vi "Sub Initialize.vi"(8 "error in (no error)":errorcluster, 11 "Instrument Recorder in":refnum<class "PID Controller.lvclass">) -> (0 "error out":errorcluster, 2 "Initialize Result":refnum<class "Acquired Result.lvclass">, 3 "Instrument Recorder out":refnum<class "PID Controller.lvclass">)   [LabVIEW 2018, in "PID Controller.lvclass"]
uses:
  PID Controller.lvclass
  C:/Program Files/National Instruments/LabVIEW 2018/vi.lib/ActorFramework/Actor/Actor.lvclass
  NHMFL_Core/Libraries/Instruments/Results/Acquired Result/Acquired Result.lvclass
  <vilib>/ActorFramework/Actor/Actor.lvclass/Actor.ctl
  <vilib>/ActorFramework/Message Enqueuer/Message Enqueuer.lvclass/Message Enqueuer.ctl
  Template Module Messages/Subscribe Request Msg/Subscribe Request Msg.lvclass/Subscribe Request Msg.ctl
  <vilib>/ActorFramework/Message Enqueuer/Init from Existing Queue.vi
  <vilib>/ActorFramework/Message Enqueuer/Enqueue.vi
  Template Module Messages/Subscribe Request Msg/Subscribe Request Msg.lvclass
  C:/Program Files/National Instruments/LabVIEW 2018/vi.lib/ActorFramework/Message/Message.lvclass
  <vilib>/ActorFramework/Message Priority Queue/Priority Enqueue.vi
  <vilib>/ActorFramework/Message Enqueuer/Message Enqueuer.lvclass
  Instrument Actor/Instrument Actor.lvclass
  <vilib>/ActorFramework/Actor/Actor.lvclass
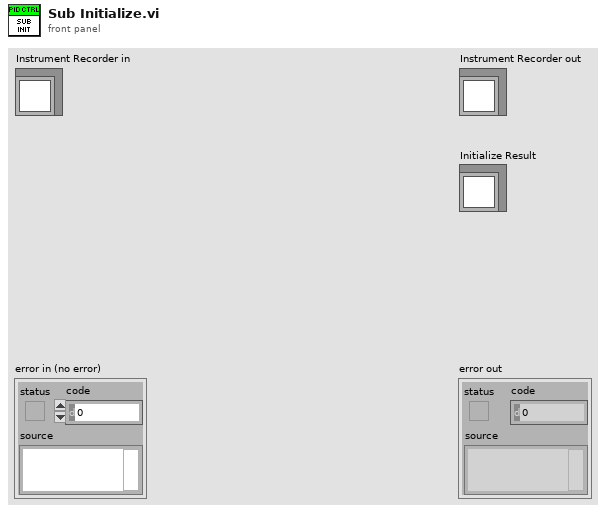
[diagram p1: front panel]
types:
  T1 = typedef "PID Controller Configuration.ctl" = cluster{"P":dbl, "I":dbl, "D":dbl, "Set point":dbl, "Input instrument":string, "Output instrument":string}
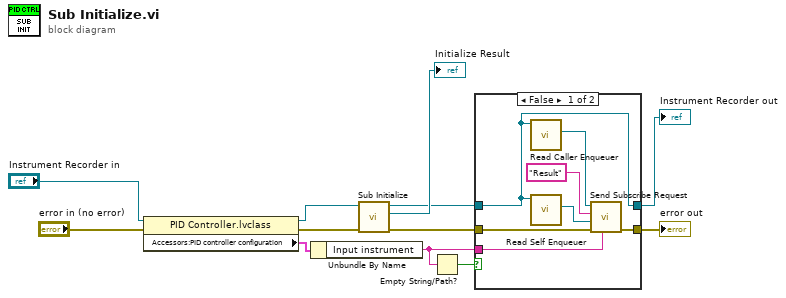
[diagram p0: block diagram]
diagram:
  n1 = property class="PID Controller.lvclass"(reference="Instrument Recorder in", error in="error in (no error)") -> (reference out=w1:refnum<class "PID Controller.lvclass">, error out=w2:errorcluster, "Accessors:PID controller configuration"=w9:T1)
  n2 = Unbundle By Name(w9) -> ("Input instrument"=w5:string)
  n3 = call-parent "Sub Initialize.vi"("error in (no error)"=w2, "Instrument Recorder in"=w1) -> ("error out"=w4:errorcluster, "Initialize Result"=→"Initialize Result":refnum<class "Acquired Result.lvclass">, "Instrument Recorder out"=w7:refnum<class "PID Controller.lvclass">)  [unwired: 7 in]
  n4 = Empty String/Path?(string/path=w5) -> (empty?=w8:bool)
  n5 = case shown="False" w8 {
    tunnel: w5 -> [w17 _]
    tunnel: w7 -> [w14 w21]
    tunnel: [w14 w21] -> w6
    tunnel: w4 -> [w19 w20]
    tunnel: [w18 w20] -> w3
    frame False {
      n6 = call <vilib>:"Read Caller Enqueuer.vi"("Actor"=w14) -> ("Caller Enqueuer"=w15:refnum<class "Message Enqueuer.lvclass">)  [unwired: 10 in]
      n7 = call <vilib>:"Read Self Enqueuer.vi"("Actor"=w14) -> ("Self Enqueuer"=w13:refnum<class "Message Enqueuer.lvclass">)  [unwired: 10 in]
      n8 = call "Send Subscribe Request.vi"("Broadcaster"=w17, "error in (no error)"=w19, "Subscriber Enqueuer"=w13, "Topic"="Result", "Message Enqueuer"=w15) -> ("error out"=w18:errorcluster)  [unwired: 5 in, 1 out]
    }
    frame True {
    }
  }
  "error out" <- w3
  "Instrument Recorder out" <- w6
